vi "INIT.vi"(8 "error in (no error)":errorcluster, 11 "UV-VIS in":refnum<class "UV-VIS.lvclass">) -> (0 "error out":errorcluster, 3 "UV-VIS out":refnum<class "UV-VIS.lvclass">)   [LabVIEW 2015, in "UV-VIS.lvclass"]
uses:
  UV-VIS.lvclass
  GeneralFunctionality/GeneralFunctionality.lvclass/GeneralFunctionality.ctl
  dependecies/AcquisitionMode_mode typedef.ctl
  methods/atmcd32d.llb/ReadMode_mode typedef.ctl
  methods/atmcd32d.llb/HSSpeed_type typedef.ctl
  methods/atmcd32d.llb/TriggerMode_mode typedef.ctl
  dependecies/ControlsVIs/Clusters-def/list-of-keys-DAQmx-tasks.ctl
  Detector.lvclass/Detector.ctl
  Config/Config.lvclass
  Detector.lvclass
  GeneralFunctionality/GeneralFunctionality.lvclass
  DAQmxTasks/DAQmxTaskContainer_General/DAQmxTaksContainer_General.lvclass
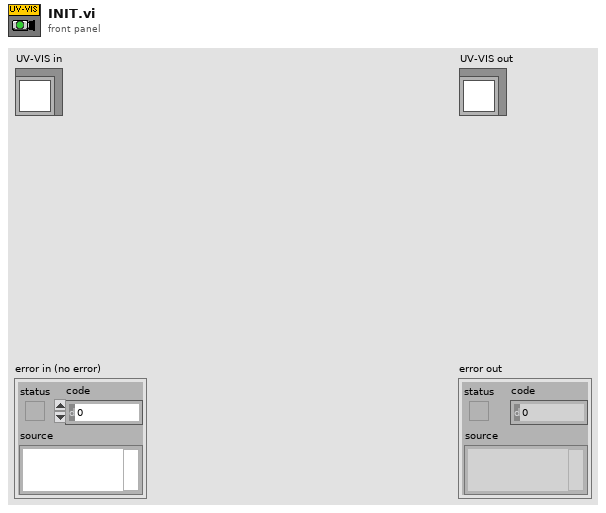
[diagram p1: front panel]
types:
  T1 = typedef "DAQmxTaksContainer_General.lvclass/list-of-keys-DAQmx-tasks.ctl" = string
  T2 = typedef "TriggerMode_mode typedef.ctl" = enum16{"Internal", "External", "N/A (2)", "N/A (3)", "N/A (4)", "N/A (5)", "External Start", "External Exposure (Bulb)", "N/A (8)", "External FVB EM", "Software", "N/A (11)", "External Charge Shifting"}
  T3 = typedef "ReadMode_mode typedef.ctl" = enum16{"Full Vertical Binning", "Multi-Track", "Random-Track", "Single-Track", "Image"}
  T4 = typedef "AcquisitionMode_mode typedef.ctl" = enum16{"Reserved (0)", "Single Scan", "Accumulate", "Kinetics", "Fast Kinetics", "Run Till Abort for non-Frame Transfer", "Frame Transfer", "Run Till Abort for Frame Transfer", "Reserved (8)", "Time Delayed Integration"}
  T5 = typedef "HSSpeed_type typedef.ctl" = enum16{"EM Amp", "Conventional Amp"}
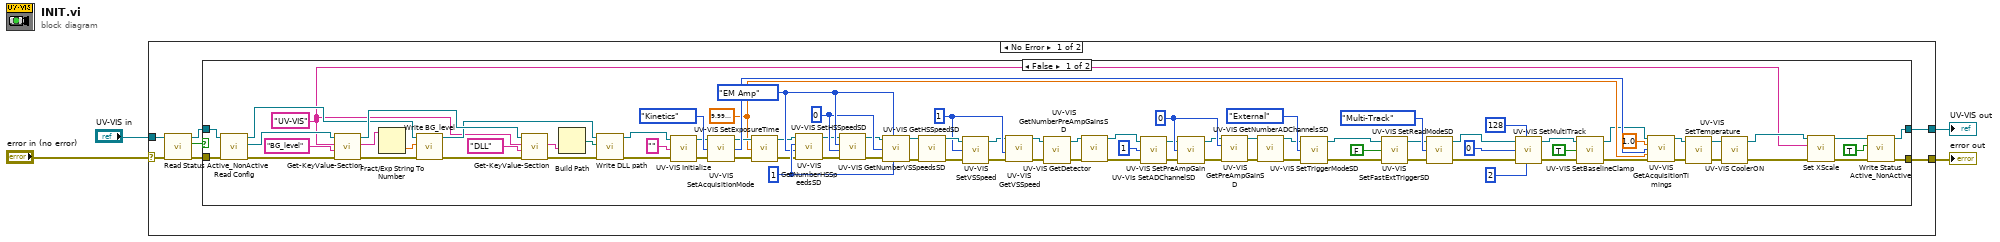
[diagram p0: block diagram]
diagram:
  n1 = case shown="No Error" "error in (no error)" {
    selector: "error in (no error)" -> [w8 w103]
    tunnel: [w5 w103] -> w4
    tunnel: [w6 w102] -> w3
    tunnel: "UV-VIS in" -> [w10 w102]
    frame No Error {
      n2 = call "Read Status Active_NonActive.vi"("error in (no error)"=w8, "GeneralFunctionality in"=w10) -> ("error out"=w7:errorcluster, "Status Active/NonActive"=w11:bool, "GeneralFunctionality out"=w9:refnum<class "UV-VIS.lvclass">)  [unwired: 7 in]
      n3 = case shown="False" w11 {
        tunnel: w7 -> [w29 w101]
        tunnel: [w39 w101] -> w5
        tunnel: [w38 w100] -> w6
        tunnel: w9 -> [w30 w100]
        frame False {
          w12 = "UV-VIS" ("Section")
          w77 = HSSpeed_type_typedef."EM Amp" ("type")
          w69 = 0 ("index HSSpeed")
          w55 = 1 ("index VSSpeed")
          w86 = 0 ("index preamp gain")
          w59 = sgl 0.0001 ("time")
          w92 = 1 ("channel HSSpeed")
          n4 = call "Read Config.vi"("error in (no error)"=w29, "GeneralFunctionality en entrée"=w30) -> ("error out"=w19:errorcluster, "Config.lvclass"=w20:refnum<class "Config.lvclass">, "GeneralFunctionality en sortie"=w15:refnum<class "UV-VIS.lvclass">)  [unwired: 7 in]
          n5 = call-dynamic "Get-KeyValue-Section.vi"("error in (no error)"=w19, "Key"="BG_level", "Section"=w12, "Config in"=w20) -> ("error out"=w21:errorcluster, "Value"=w23:string, "Config out"=w18:refnum<class "Config.lvclass">)  [unwired: 5 in]
          n6 = Fract/Exp String To Number(string=w23) -> (number=w24:dbl)  [unwired: 3 in, 1 out]
          n7 = call-dynamic "Write BG_level.vi"("error in (no error)"=w21, "BG_level"=w24, "Detector in"=w15) -> ("error out"=w13:errorcluster, "Detector out"=w14:refnum<class "UV-VIS.lvclass">)  [unwired: 7 in]
          n8 = call-dynamic "Get-KeyValue-Section.vi"("error in (no error)"=w13, "Key"=T1 "DLL", "Section"=w12, "Config in"=w18) -> ("error out"=w25:errorcluster, "Value"=w26:string)  [unwired: 5 in, 1 out]
          n9 = Build Path(name or relative path=w26) -> (appended path=w28:path)  [unwired: 1 in]
          n10 = call "Write DLL path.vi"("error in (no error)"=w25, "DLL path"=w28, "Detector in"=w14) -> ("error out"=w16:errorcluster, "Detector out"=w17:refnum<class "UV-VIS.lvclass">)  [unwired: 7 in]
          n11 = call "UV-VIS Initialize.vi"("error in (no error)"=w16, "directory (\"\")"="" ("directory (\"\")"), "UV-VIS in"=w17) -> ("error out"=w67:errorcluster, "Control out"=w64:refnum<class "UV-VIS.lvclass">)  [unwired: 1 out]
          n12 = call "UV-VIS SetAcquisitionMode.vi"("error in (no error)"=w67, "mode"=AcquisitionMode_mode_typedef."Kinetics", "Control in"=w64) -> ("error out"=w72:errorcluster, "DLL error code"=w73:u32, "Control out"=w63:refnum<class "UV-VIS.lvclass">)
          n13 = call "UV-VIS SetExposureTime.vi"("error in (no error)"=w72, "time"=w59, "Control in"=w63) -> ("error out"=w84:errorcluster, "Control out"=w62:refnum<class "UV-VIS.lvclass">)  [unwired: 1 out]
          n14 = call "UV-VIS GetNumberHSSpeedsSD.vi"("error in (no error)"=w84, "type"=w77, "channel"=w92, "Control in"=w62) -> ("error out"=w93:errorcluster, "Control out"=w61:refnum<class "UV-VIS.lvclass">)  [unwired: 2 out]
          n15 = call "UV-VIS SetHSSpeedSD.vi"("error in (no error)"=w93, "index"=w69, "type"=w77, "Control in"=w61) -> ("error out"=w94:errorcluster, "Control out"=w60:refnum<class "UV-VIS.lvclass">)  [unwired: 1 in, 1 out]
          n16 = call "UV-VIS GetHSSpeedSD.vi"("Control in"=w60, "type"=w77, "index"=w69, "error in (no error)"=w94, "channel"=w92) -> ("Control out"=w57:refnum<class "UV-VIS.lvclass">, "error out"=w83:errorcluster)  [unwired: 2 out]
          n17 = call "UV-VIS GetNumberVSSpeedsSD.vi"("error in (no error)"=w83, "Control in"=w57) -> ("error out"=w91:errorcluster, "Control out"=w56:refnum<class "UV-VIS.lvclass">)  [unwired: 2 in, 2 out]
          n18 = call "UV-VIS SetVSSpeed.vi"("error in (no error)"=w91, "index"=w55, "Control in"=w56) -> ("error out"=w90:errorcluster, "Control out"=w54:refnum<class "UV-VIS.lvclass">)  [unwired: 1 out]
          n19 = call "UV-VIS GetVSSpeed.vi"("error in (no error)"=w90, "index"=w55, "Control in"=w54) -> ("error out"=w82:errorcluster, "Control out"=w52:refnum<class "UV-VIS.lvclass">)  [unwired: 1 in, 2 out]
          n20 = call "UV-VIS GetDetector.vi"("UV-VIS in"=w52, "error in (no error)"=w82) -> ("UV-VIS out"=w40:refnum<class "UV-VIS.lvclass">, "error out"=w81:errorcluster)  [unwired: 3 in, 3 out]
          n21 = call "UV-VIS GetNumberPreAmpGainsSD.vi"("error in (no error)"=w81, "UV-VIS in"=w40) -> ("error out"=w71:errorcluster, "UV-VIS out"=w51:refnum<class "UV-VIS.lvclass">)  [unwired: 2 in, 2 out]
          n22 = call "UV-VIs SetADChannelSD.vi"("error in (no error)"=w71, "channel"=1, "Control in"=w51) -> ("error out"=w70:errorcluster, "Control out"=w53:refnum<class "UV-VIS.lvclass">)  [unwired: 1 out]
          n23 = call "UV-VIS SetPreAmpGain.vi"("error in (no error)"=w70, "index"=w86, "Control in"=w53) -> ("error out"=w96:errorcluster, "Control out"=w49:refnum<class "UV-VIS.lvclass">)  [unwired: 1 out]
          n24 = call "UV-VIS GetPreAmpGainSD.vi"("error in (no error)"=w96, "index"=w86, "Control in"=w49) -> ("error out"=w76:errorcluster, "Control out"=w48:refnum<class "UV-VIS.lvclass">)  [unwired: 1 in, 2 out]
          n25 = call "UV-VIS GetNumberADChannelsSD.vi"("error in (no error)"=w76, "Control in"=w48) -> ("error out"=w80:errorcluster, "Control out"=w46:refnum<class "UV-VIS.lvclass">)  [unwired: 2 in, 2 out]
          n26 = call "UV-VIS SetTriggerModeSD.vi"("error in (no error)"=w80, "mode"=TriggerMode_mode_typedef."External", "Control in"=w46) -> ("error out"=w99:errorcluster, "Control out"=w45:refnum<class "UV-VIS.lvclass">)  [unwired: 1 out]
          n27 = call "UV-VIS SetFastExtTriggerSD.vi"("error in (no error)"=w99, "mode"=FALSE ("Fast external mode"), "Control in"=w45) -> ("error out"=w79:errorcluster, "Control out"=w47:refnum<class "UV-VIS.lvclass">)  [unwired: 1 out]
          n28 = call "UV-VIS SetReadModeSD.vi"("error in (no error)"=w79, "mode"=ReadMode_mode_typedef."Multi-Track" ("readout  mode"), "Control in"=w47) -> ("error out"=w95:errorcluster, "Control out"=w50:refnum<class "UV-VIS.lvclass">)  [unwired: 1 out]
          n29 = call "UV-VIS SetMultiTrack.vi"("Control in"=w50, "height"=128, "offset"=0, "error in (no error)"=w95, "number"=2) -> ("Control out"=w32:refnum<class "UV-VIS.lvclass">, "error out"=w66:errorcluster)  [unwired: 3 out]
          n30 = call "UV-VIS SetBaselineClamp.vi"("error in (no error)"=w66, "state"=TRUE ("Base line Clamp"), "Control in"=w32) -> ("error out"=w65:errorcluster, "Control out"=w58:refnum<class "UV-VIS.lvclass">)  [unwired: 1 out]
          n31 = call "UV-VIS GetAcquisitionTimings.vi"("Control in"=w58, "accumulate input"=sgl 1.0, "kinetic input"=w73, "exposure input"=w59, "error in (no error)"=w65) -> ("Control out"=w44:refnum<class "UV-VIS.lvclass">, "error out"=w43:errorcluster)  [unwired: 5 in, 4 out]
          n32 = call "UV-VIS SetTemperature.vi"("error in (no error)"=w43, "UV-VIS detector in"=w44) -> ("error out"=w42:errorcluster, "UV-VIS detector out"=w41:refnum<class "UV-VIS.lvclass">)  [unwired: 1 in, 1 out]
          n33 = call "UV-VIS CoolerON.vi"("error in (no error)"=w42, "UV-VIS  in"=w41) -> ("error out"=w36:errorcluster, "UV-VIS  out"=w37:refnum<class "UV-VIS.lvclass">)  [unwired: 1 in, 1 out]
          n34 = call "Set XScale.vi"("error in (no error)"=w36, "Section"=w12, "Detector en entrée"=w37) -> ("error out"=w33:errorcluster, "Detector en sortie"=w34:refnum<class "UV-VIS.lvclass">)  [unwired: 7 in]
          n35 = call "Write Status Active_NonActive.vi"("error in (no error)"=w33, "Status Active/NonActive"=TRUE, "GeneralFunctionality in"=w34) -> ("error out"=w39:errorcluster, "GeneralFunctionality out"=w38:refnum<class "UV-VIS.lvclass">)  [unwired: 7 in]
        }
        frame True {
        }
      }
    }
    frame Error {
    }
  }
  "error out" <- w4
  "UV-VIS out" <- w3
